vi "Write.vi"(8 "error in":errorcluster, 10 "Data In":string, 11 "Text Session in":refnum<class "FPGA Serial Session.lvclass">) -> (0 "error out":errorcluster, 3 "Text Session out":refnum<class "FPGA Serial Session.lvclass">)   [LabVIEW 2015, in "FPGA Serial Session.lvclass"]
uses:
  FPGA Serial Session.lvclass
  FPGA Serial Session.lvclass/FPGA Serial Session.ctl
  Raw FPGA/FPGA Session.lvclass
  FPGA/Serial Data In.ctl
  Raw FPGA/FPGA Session.lvclass/FPGA Session.ctl
  Raw FPGA/Read FPGA Ref.vi
  <vilib>/rvi/errors/niLvFpgaAdjustHostInterfaceError.vi
  <vilib>/RVI Host/nirviSupport.llb/nirviErrorClusterFromErrorCode.vi
  <vilib>/Utility/error.llb/Error Cluster From Error Code.vi
  FPGA Ref.ctl
  <vilib>/rvi/interface/nirviMethod/nirviMethod.xnode
  FPGA Bitfiles/NickIO.lvbitx
  <vilib>/rvi/interface/nirviReadWriteControl/nirviReadWriteControl.xnode
  NiFpgaLv.dll
  <vilib>/FPGAPlugInAG/cRIO-9081/niLvFpga_AcknowledgeIrq_cRIO-9081.vi
  <vilib>/rvi/interface/nirviMethod/StockFPGA_InlinedMethodWaitForSingleIRQ.vi
  <vilib>/FPGAPlugInAG/cRIO-9081/niLvFpga_WaitOnIrq_cRIO-9081.vi
panel:
  out "IRQ Timeout":bool
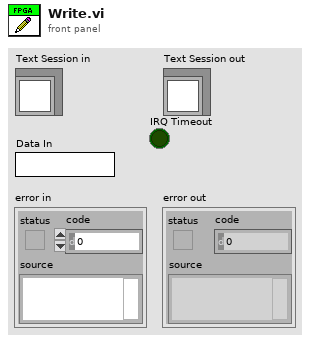
[diagram p1: front panel]
types:
  T1 = typedef "Serial Data In.ctl" = cluster{"Data":u8[], "NumBytes":i32, "RS485_Cmd":enum8{"Read", "Write", "Idle"}, "Timeout (ms)":i32}
  T2 = typedef "Session - Root.lvclass/Session Handle.ctl" = refnum<data-value>
  T3 = enum16{"Port 1", "Port 2", "Port 3", "Port 4", "None"}
  T4 = typedef "FPGA Ref.ctl" = refnum<k20>
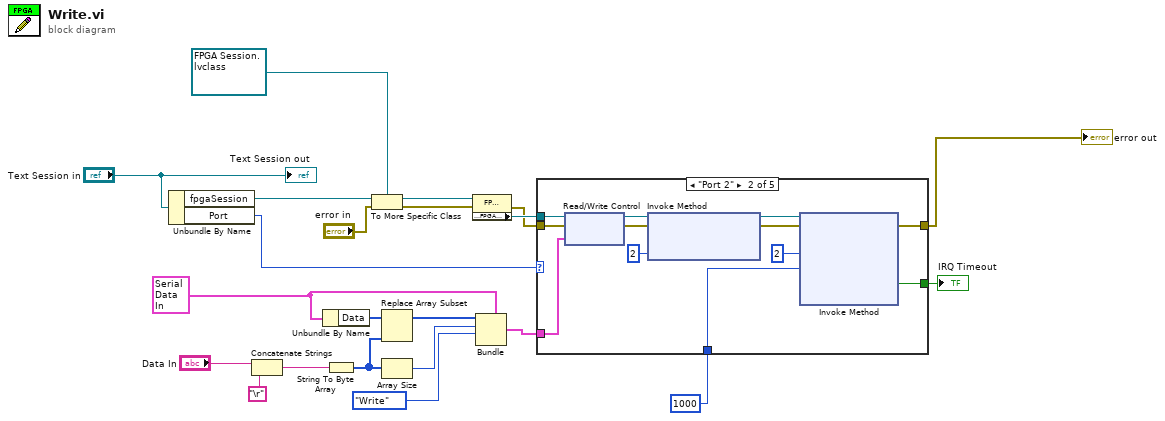
[diagram p0: block diagram]
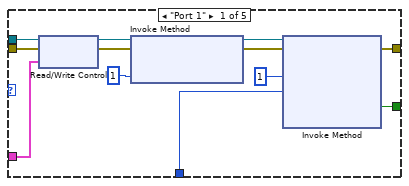
[diagram p2: hidden frame]
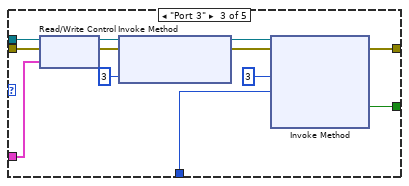
[diagram p3: hidden frame]
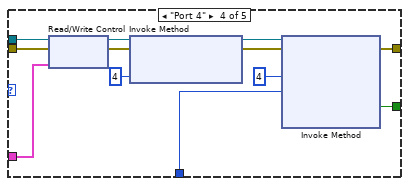
[diagram p4: hidden frame]
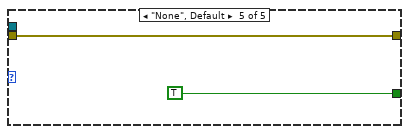
[diagram p5: hidden frame]
diagram:
  w3 = T1 {"Data"=[0, 0, 0, 0, 0, 0, 0, 0, 0, 0, 0, 0, 0, 0, 0, 0, 0, 0, 0, 0], "NumBytes"=0, "RS485_Cmd"=enum."Read", "Timeout (ms)"=1000} ("Port3 In")
  n1 = Unbundle By Name("Text Session in") -> ("fpgaSession"=w21:T2, "Port"=w7:T3)
  n2 = Concatenate Strings("Data In", "\r") -> (w13:string)
  n3 = Unbundle By Name(w3) -> ("Data"=w9:u8[])
  n4 = String To Byte Array(string=w13) -> (unsigned byte array=w11:u8[])
  n5 = To More Specific Class(target class=refnum<data-value> refnum ("fpgaSession"), reference=w21, error in="error in") -> (specific class reference=w19:refnum<data-value>, error out=w18:errorcluster)
  n6 = Replace Array Subset(array=w9, new element=w11) -> (w10:u8[])  [unwired: 1 in]
  n7 = Array Size(array=w11) -> (size(s)=w12:i32)
  n8 = property class="FPGA Session"(reference=w19, error in=w18) -> (error out=w15:errorcluster, "Accessors:FPGA Ref"=w16:T4)  [unwired: 1 out]
  n9 = Bundle(cluster=w3, "Data"=w10, "NumBytes"=w12, "RS485_Cmd"=enum8{"Read", "Write", "Idle"}."Write") -> (w6:T1)  [unwired: 1 in]
  n10 = case shown="\"Port 2\"" w7 {
    tunnel: w16 -> [w34 w46 w58 w70 _]
    tunnel: w15 -> [w33 w45 w57 w69 w72]
    tunnel: w6 -> [w27 w38 w47 w62 _]
    tunnel: [w25 w37 w50 w61 w72] -> w1
    tunnel: [w24 w36 w49 w60 TRUE ("Timed Out")] -> w5
    tunnel: 1000 ("Timeout (ms)") -> [w23 w35 w48 w59 _]
    frame "Port 1" {
      n11 = xnode "Read/Write Control"("FPGA VI Reference In"=w34, "error in"=w33, "Port1 In"=w27) -> ("FPGA VI Reference Out"=w28:T4, "error out"=w26:errorcluster)
      n12 = xnode "Invoke Method"("FPGA VI Reference In"=w28, "error in"=w26, "IRQ Number(s)"=1) -> ("FPGA VI Reference Out"=w30:T4, "error out"=w31:errorcluster)
      n13 = xnode "Invoke Method"("FPGA VI Reference In"=w30, "error in"=w31, "IRQ Number(s)"=1, "Timeout (ms)"=w23) -> ("error out"=w25:errorcluster, "Timed Out"=w24:bool)  [unwired: 2 out]
    }
    frame "Port 2" {
      n14 = xnode "Read/Write Control"("FPGA VI Reference In"=w46, "error in"=w45, "Port2 In"=w38) -> ("FPGA VI Reference Out"=w40:T4, "error out"=w39:errorcluster)
      n15 = xnode "Invoke Method"("FPGA VI Reference In"=w40, "error in"=w39, "IRQ Number(s)"=2) -> ("FPGA VI Reference Out"=w42:T4, "error out"=w43:errorcluster)
      n16 = xnode "Invoke Method"("FPGA VI Reference In"=w42, "error in"=w43, "IRQ Number(s)"=2, "Timeout (ms)"=w35) -> ("error out"=w37:errorcluster, "Timed Out"=w36:bool)  [unwired: 2 out]
    }
    frame "Port 3" {
      n17 = xnode "Read/Write Control"("FPGA VI Reference In"=w58, "error in"=w57, "Port3 In"=w47) -> ("FPGA VI Reference Out"=w52:T4, "error out"=w51:errorcluster)
      n18 = xnode "Invoke Method"("FPGA VI Reference In"=w52, "error in"=w51, "IRQ Number(s)"=3) -> ("FPGA VI Reference Out"=w54:T4, "error out"=w55:errorcluster)
      n19 = xnode "Invoke Method"("FPGA VI Reference In"=w54, "error in"=w55, "IRQ Number(s)"=3, "Timeout (ms)"=w48) -> ("error out"=w50:errorcluster, "Timed Out"=w49:bool)  [unwired: 2 out]
    }
    frame "Port 4" {
      n20 = xnode "Read/Write Control"("FPGA VI Reference In"=w70, "error in"=w69, "Port4 In"=w62) -> ("FPGA VI Reference Out"=w64:T4, "error out"=w63:errorcluster)
      n21 = xnode "Invoke Method"("FPGA VI Reference In"=w64, "error in"=w63, "IRQ Number(s)"=4) -> ("FPGA VI Reference Out"=w66:T4, "error out"=w67:errorcluster)
      n22 = xnode "Invoke Method"("FPGA VI Reference In"=w66, "error in"=w67, "IRQ Number(s)"=4, "Timeout (ms)"=w59) -> ("error out"=w61:errorcluster, "Timed Out"=w60:bool)  [unwired: 2 out]
    }
    frame "None", Default {
    }
  }
  "error out" <- w1
  "IRQ Timeout" <- w5
  "Text Session out" <- "Text Session in"
